vi "SplineHelp_GetQuinticCtrlVectorsFromWayPts_2762.vi"(11 "WayPoints":T1[](array[typedef]) {"ROTATION"."SIN" format="%13.4f"; "ROTATION"."COS" format="%13.4f"; "ROTATION"."VALUE" format="%13.4f"; "TRANSLATION"."Y" format="%14.3f"; "TRANSLATION"."X" format="%14.3f"}) -> (3 "SplineControlVectors":T4[](array[typedef]))   [LabVIEW 2019]
doc: "Returns quintic control vectors from a set of waypoints.\n\nParameters:\n - waypoints - The array of waypoints (Translation)\n\nReturns:\n - SplineControlVectors - Array of control vectors"
uses:
  SPLINE_CTRL_VECTOR.ctl
  POSE2D.ctl
  TRANSLATION2D.ctl
  ROTATION2D.ctl
  Util_CalcDist.vi
  Trajectory_Library.lvlib
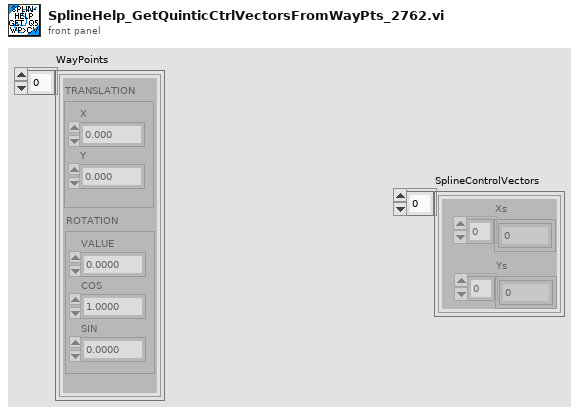
[diagram p1: front panel]
types:
  T1 = typedef "Trajectory_Library.lvlib/POSE2D.ctl" = cluster{"TRANSLATION":T2, "ROTATION":T3}
  T2 = typedef "Trajectory_Library.lvlib/TRANSLATION2D.ctl" = cluster{"X":dbl, "Y":dbl}
  T3 = typedef "Trajectory_Library.lvlib/ROTATION2D.ctl" = cluster{"VALUE":dbl, "COS":dbl, "SIN":dbl}
  T4 = typedef "Trajectory_Library.lvlib/SPLINE_CTRL_VECTOR.ctl" = cluster{"Xs":dbl[], "Ys":dbl[]}
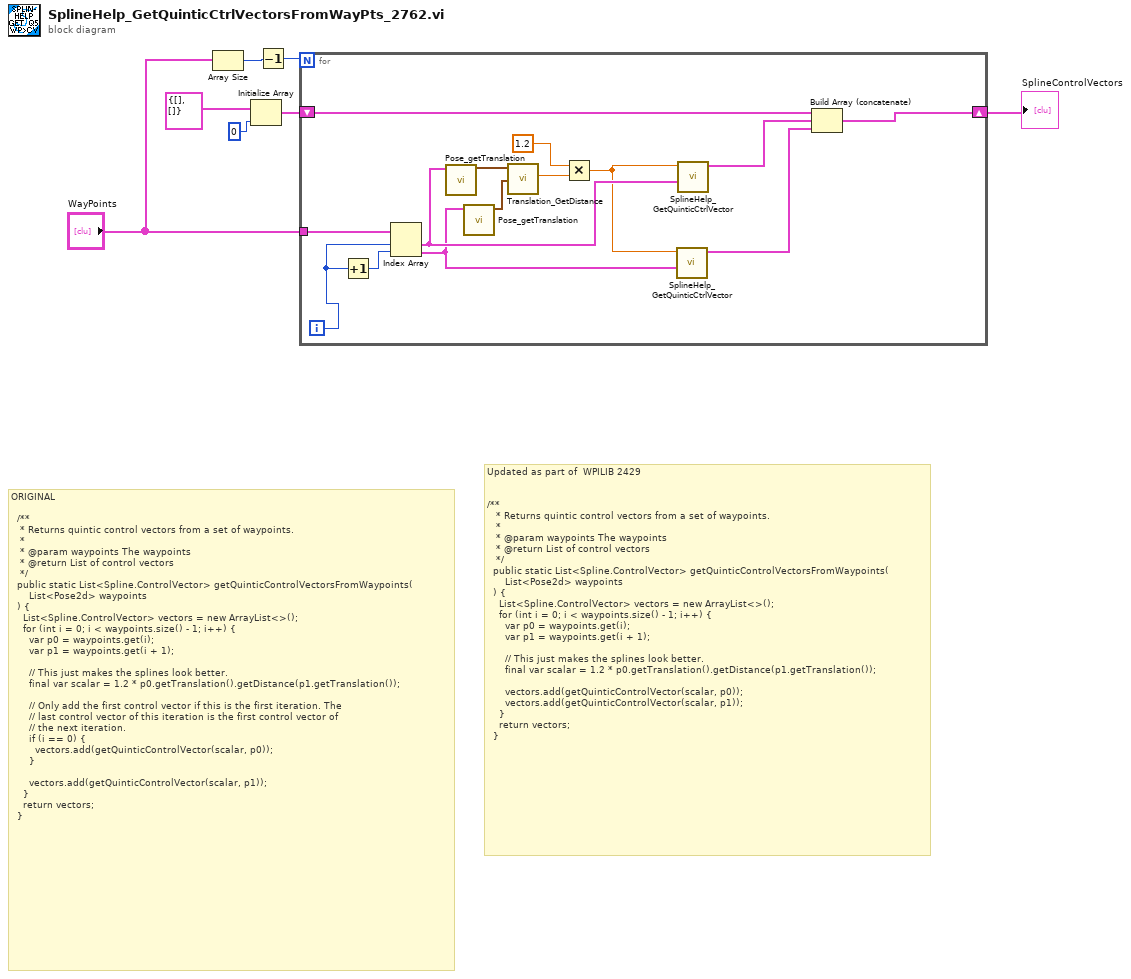
[diagram p0: block diagram]
diagram:
  # "Updated as part of  WPILIB 2429 \n\n\n/**\n   * Returns quintic control vectors from a set of waypoints.\n   *\n   * @param waypoints The waypoints\n   * @return List of control vectors\n   */\n  public static List<Spline.ControlVector> getQuinticControlVectorsFromWaypoints(\n      List<Pose2d> waypoints\n  ) {\n    List<Spline.ControlVector> vectors = new ArrayList<>();\n    for (int i = 0; i < waypoints.size() - 1; i++) {\n      var p0 = waypoints.get(i);\n      var p1 = waypoints.get(i + 1);\n\n      // This just makes the splines look better.\n      final var scalar = 1.2 * p0.getTranslation().getDistance(p1.getTranslation());\n\n      vectors.add(getQuinticControlVector(scalar, p0));\n      vectors.add(getQuinticControlVector(scalar, p1));\n    }\n    return vectors;\n  }"
  # "ORIGINAL \n\n  /**\n   * Returns quintic control vectors from a set of waypoints.\n   *\n   * @param waypoints The waypoints\n   * @return List of control vectors\n   */\n  public static List<Spline.ControlVector> getQuinticControlVectorsFromWaypoints(\n      List<Pose2d> waypoints\n  ) {\n    List<Spline.ControlVector> vectors = new ArrayList<>();\n    for (int i = 0; i < waypoints.size() - 1; i++) {\n      var p0 = waypoints.get(i);\n      var p1 = waypoints.get(i + 1);\n\n      // This just makes the splines look better.\n      final var scalar = 1.2 * p0.getTranslation().getDistance(p1.getTranslation());\n\n      // Only add the first control vector if this is the first iteration. The\n      // last control vector of this iteration is the first control vector of\n      // the next iteration.\n      if (i == 0) {\n        vectors.add(getQuinticControlVector(scalar, p0));\n      }\n\n      vectors.add(getQuinticControlVector(scalar, p1));\n    }\n    return vectors;\n  }"
  n1 = Array Size(array="WayPoints") -> (size(s)=w6:i32)
  n2 = Initialize Array(T4 {"Xs"=[], "Ys"=[]} ("SPLINE_CTRL_VECTOR"), 0 ("dimension size")) -> (w3:T4[])
  n3 = Decrement(x=w6) -> (x-1=w7:i32)
  n4 = for {
    N: w7 -> [_]
    tunnel: "WayPoints" -> [w19]
    shift-right: [w8] -> w1
    shift-left: w3 -> [w14]
    i -> [w11]
    n5 = Increment(x=w11) -> (x+1=w20:i32)
    n6 = Index Array(array=w19, index #1=w11, index #2=w20) -> (element #1=w16:T1, element #2=w12:T1)
    n7 = call "Pose_getTranslation.vi"("in POSE"=w16) -> ("outTRANSLATION"=w17:T2)  [unwired: 10 in]
    n8 = call "Pose_getTranslation.vi"("in POSE"=w12) -> ("outTRANSLATION"=w15:T2)  [unwired: 10 in]
    n9 = call "Translation_GetDistance.vi"("other Translation"=w15, "In Translation"=w17) -> ("Distance"=w18:dbl)  [unwired: 9 in]
    n10 = Multiply(x=1.2, y=w18) -> (x*y=w13:dbl)
    n11 = call "SplineHelp_GetQuinticCtrlVector.vi"("Input POSE"=w12, "Scalar"=w13) -> ("resultSpline_Ctrl_Vector"=w9:T4)  [unwired: 9 in]
    n12 = call "SplineHelp_GetQuinticCtrlVector.vi"("Input POSE"=w16, "Scalar"=w13) -> ("resultSpline_Ctrl_Vector"=w10:T4)  [unwired: 9 in]
    n13 = Build Array (concatenate)(w14, w10, w9) -> (w8:T4[])
  }
  "SplineControlVectors" <- w1
